vi "Aquire Continuous Anolog Data..vi"() -> ()   [LabVIEW 2020]
uses:
  <instrlib>/BDAQ-6104/Public/Data/Read Single Analog Channel.vi
  <instrlib>/BDAQ-6104/BDAQ-6104.lvlib
panel:
  out "Waveform Chart":dbl(graph)
  in  "stop":bool
  in  "Channel":T1(ring)
  in  "VISA resource name":refnum<visa-resource-name>
  # "Aquire continuous channel data. Default value is in volts."
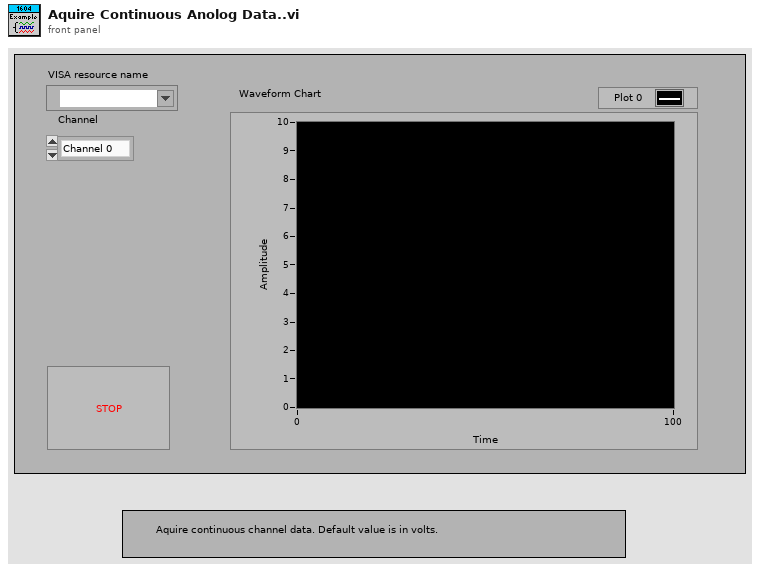
[diagram p1: front panel]
types:
  T1 = enum16{"Channel 0", "Channel 1", "Channel 2", "Channel 3", "Channel 4", "Channel 5"}
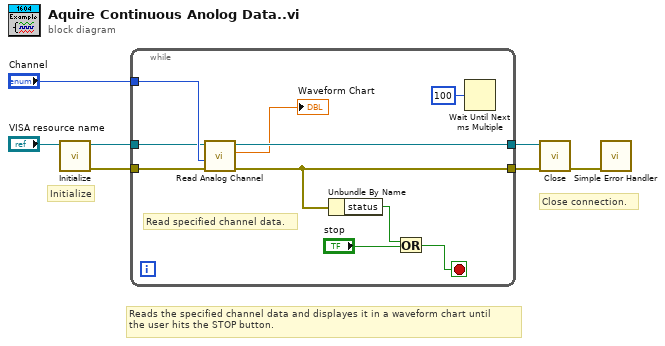
[diagram p0: block diagram]
diagram:
  # "Reads the specified channel data and displayes it in a waveform chart until\nthe user hits the STOP button."
  # "Close connection."
  # "Initialize"
  n1 = call <instrlib>:"Initialize.vi"("VISA resource name"="VISA resource name") -> ("error out"=w5:errorcluster, "VISA resource name out"=w6:refnum<visa-resource-name>)  [unwired: 9 in]
  n2 = while {
    tunnel: w6 -> [w15]
    tunnel: w5 -> [w17]
    tunnel: "Channel" -> [w16]
    tunnel: [w14] -> w3
    tunnel: [w13] -> w2
    stop <- w12 stop-if-true
    # "Read specified channel data."
    n3 = call-poly <instrlib>:"Read Analog Channel.vi"("error in (no error)"=w17, "Channel"=w16, "VISA resource name"=w15) -> ("error out"=w13:errorcluster, "Channel Data"=→"Waveform Chart":dbl, "VISA resource name"=w14:refnum<visa-resource-name>)  [unwired: 6 in]
    n4 = Unbundle By Name(w13) -> ("status"=w11:bool)
    n5 = Or(x=w11, y="stop") -> (x .or. y?=w12:bool)
    n6 = Wait Until Next ms Multiple(millisecond multiple=u32 100) -> ()  [unwired: 1 out]
  }
  n7 = call <instrlib>:"Close.vi"("error in (no error)"=w2, "VISA resource name"=w3) -> ("error out"=w1:errorcluster)  [unwired: 9 in]
  n8 = call <vilib>:"Simple Error Handler.vi"("error in (no error)"=w1) -> ()  [unwired: 4 in, 5 out]
